vi "Calculator.vi"() -> ()   [LabVIEW 2013]
doc: "This VI is a fully-functional calculator built in LabVIEW. It demonstrates the following concepts taught in the LabVIEW Basics class.\n\n- Dataflow Programming\n- Modular Programming\n- While Loops\n- Shift Registers\n- Case Structures\n- Functional Global Variables\n- Event-Driven Programming\n- VI Documentation\n- Control/Indicator Documentation\n- Custom Controls/Type Definitions\n- LabVIEW Project and Application Builder\n\nAuthor: Erik Johnson, National Instruments"
panel:
  out "Output":string
  in  "Input":string
  in  "error in (no error)":errorcluster
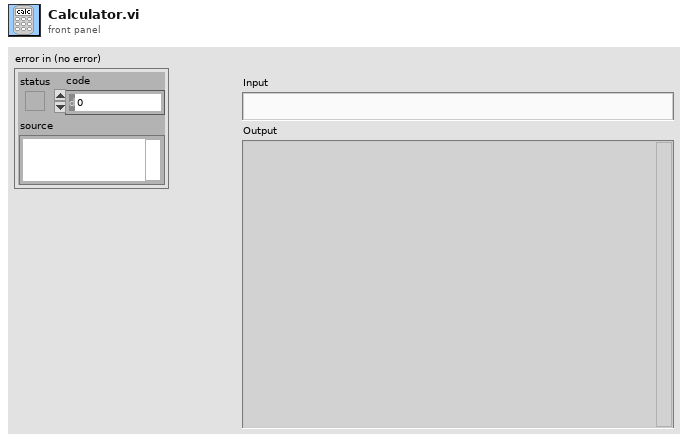
[diagram p1: front panel]
types:
  T1 = typedef "eventvkey.ctl" = enum16{"ASCII", "Enter", "Return", "Shift", "Ctrl", "Alt", "Cmd", "Opt", "Caps", "NumLock", "Clear", "Break", "Up", "Down", "Left", "Right", "Insert", "Delete", "Home", "End", "PageUp", "PageDown", "Escape", "Help", "Pause", "ScrollLock", "F1", "F2", "F3", "F4", "F5", "F6", "F7", "F8", "F9", "F10", "F11", "F12", "F13", "F14", "F15", "F16", "F17", "F18", "F19", "F20", "F21", "F22", "F23", "F24", "Play", "VolumeUp", "VolumeDown", "Mute", "Two Byte Char"}
  T2 = enum32{"invalid app kind", "Development System", "Run Time System", "Student Edition", "Embedded LabVIEW", "Evaluation", "Custom"}
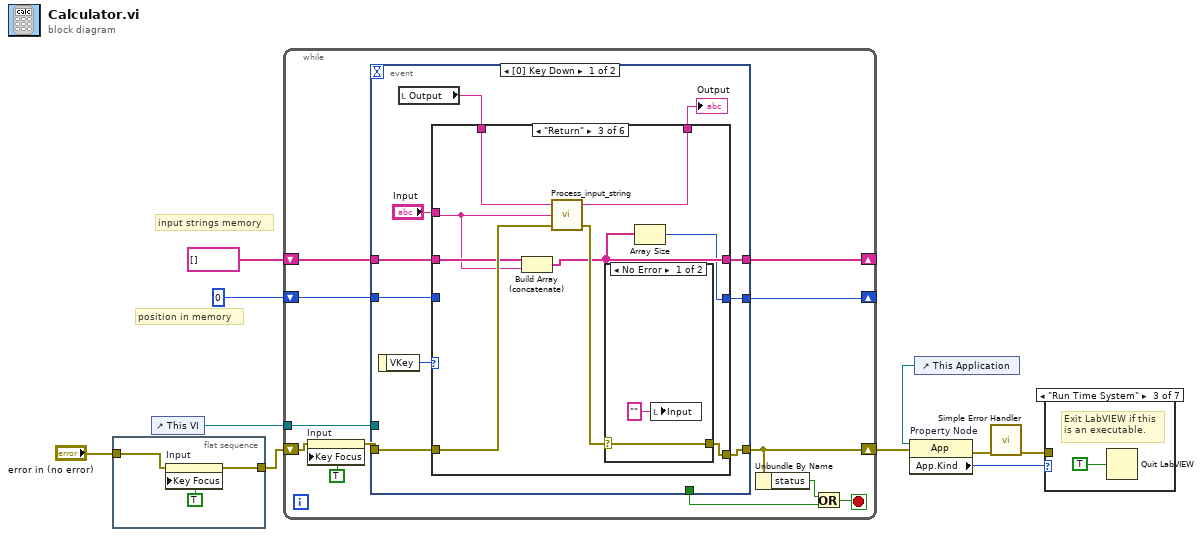
[diagram p0: block diagram]
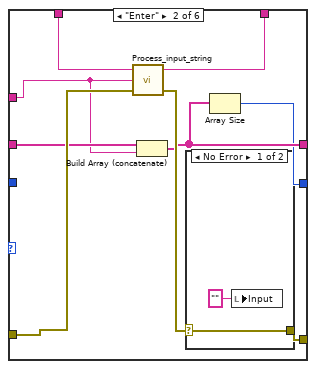
[diagram p9: hidden frame]
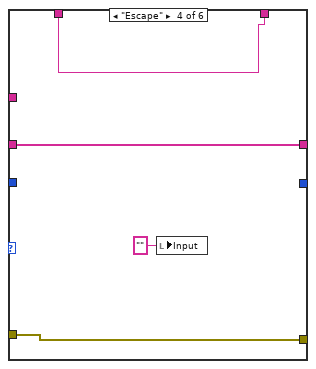
[diagram p12: hidden frame]
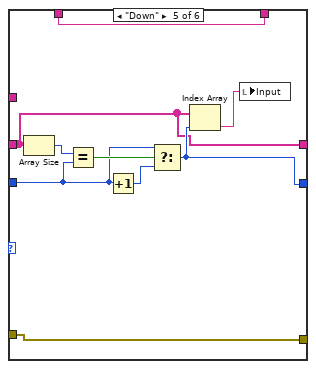
[diagram p13: hidden frame]
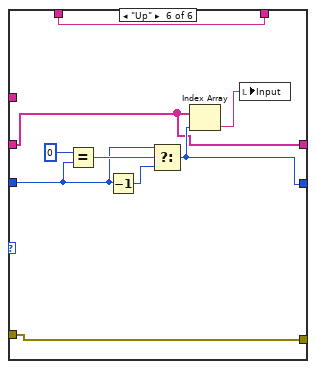
[diagram p14: hidden frame]
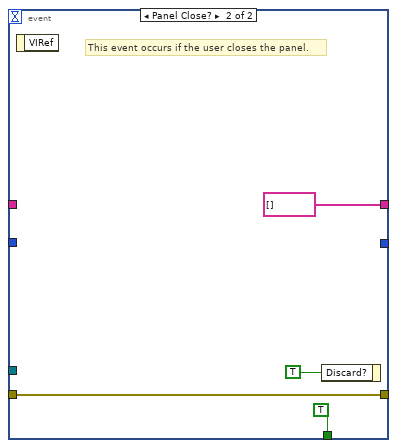
[diagram p15: hidden frame]
diagram:
  # "position in memory"
  # "input strings memory"
  n1 = flat-sequence {
    tunnel: "error in (no error)" -> [w12]
    tunnel: [w11] -> w1
    frame #0 {
      n2 = property on="Input" class="Str"(error in=w12, "Key Focus"=TRUE) -> (error out=w11:errorcluster)  [unwired: 1 in, 1 out]
    }
  }
  n3 = control-ref of="This VI"() -> (w5:refnum<vi>)
  n4 = while {
    tunnel: w5 -> [w25]
    shift-right: [w23] -> w6
    shift-left: w1 -> [w15]
    shift-right: [w19] -> _
    shift-left: string[] [] -> [w20]
    shift-right: [w17] -> _
    shift-left: 0 -> [w18]
    stop <- w24 stop-if-true
    n5 = property on="Input" class="Str"(error in=w15, "Key Focus"=TRUE) -> (error out=w14:errorcluster)  [unwired: 1 in, 1 out]
    n6 = event shown="[0] Key Down" {
      selector: _ -> [_ _]
      dyn-events: _ -> [_ _]
      timeout: _ -> [_ _]
      tunnel: [_ TRUE ("Discard?")] -> w21
      tunnel: w25 -> [_ _]
      tunnel: w14 -> [w31 w86]
      tunnel: [w30 w86] -> w23
      tunnel: w20 -> [w29 _]
      tunnel: [w28 string[] []] -> w19
      tunnel: w18 -> [w27 _]
      tunnel: [w26 _] -> w17
      event Key Down {
        n7 = event-data() -> ("VKey"=w35:T1)  [unwired: 1 in]
        n8 = local read "Output"() -> (w33:string)
        n9 = case shown="\"Return\"" w35 {
          tunnel: "Input" -> [_ w43 w55 _ _ _]
          tunnel: w33 -> [w38 w47 w58 w65 w68 w77]
          tunnel: [w38 w46 w59 w65 w68 w77] -> w32
          tunnel: w31 -> [w37 w45 w57 w64 w67 w76]
          tunnel: [w37 w41 w53 w64 w67 w76] -> w30
          tunnel: w29 -> [w36 w44 w56 w63 w69 w79]
          tunnel: [w36 w40 w52 w63 w69 w79] -> w28
          tunnel: w27 -> [_ _ _ _ w73 w83]
          tunnel: [_ w39 w51 _ w71 w81] -> w26
          frame "ASCII", Default {
          }
          frame "Enter" {
            n10 = call "Process_input_string.vi"("error in (no error)"=w45, "Input"=w43, "Output_window_old"=w47) -> ("error out"=w42:errorcluster, "Output"=w46:string)  [unwired: 1 out]
            n11 = Build Array (concatenate)(w44, w43) -> (w40:string[])
            n12 = case shown="No Error" w42 {
              selector: w42 -> [w49 w50]
              tunnel: [w49 w50] -> w41
              frame No Error {
                n13 = local write "Input"("" ("Input")) -> ()
              }
              frame Error {
              }
            }
            n14 = Array Size(array=w40) -> (size(s)=w39:i32)
          }
          frame "Return" {
            n15 = Build Array (concatenate)(w56, w55) -> (w52:string[])
            n16 = call "Process_input_string.vi"("error in (no error)"=w57, "Input"=w55, "Output_window_old"=w58) -> ("error out"=w54:errorcluster, "Output"=w59:string)  [unwired: 1 out]
            n17 = case shown="No Error" w54 {
              selector: w54 -> [w61 w62]
              tunnel: [w61 w62] -> w53
              frame No Error {
                n18 = local write "Input"("" ("Input")) -> ()
              }
              frame Error {
              }
            }
            n19 = Array Size(array=w52) -> (size(s)=w51:i32)
          }
          frame "Escape" {
            n20 = local write "Input"("" ("Input")) -> ()
          }
          frame "Down" {
            n21 = Array Size(array=w69) -> (size(s)=w75:i32)
            n22 = Equal?(x=w75, y=w73) -> (x = y?=w74:bool)
            n23 = Increment(x=w73) -> (x+1=w72:i32)
            n24 = Select(t=w73, s=w74, f=w72) -> (s? t:f=w71:i32)
            n25 = Index Array(array=w69, index=w71) -> (element=w70:string)
            n26 = local write "Input"(w70) -> ()
          }
          frame "Up" {
            n27 = Equal?(x=0, y=w83) -> (x = y?=w84:bool)
            n28 = Decrement(x=w83) -> (x-1=w82:i32)
            n29 = Select(t=w83, s=w84, f=w82) -> (s? t:f=w81:i32)
            n30 = Index Array(array=w79, index=w81) -> (element=w80:string)
            n31 = local write "Input"(w80) -> ()
          }
        }
        "Output" <- w32
      }
      event Panel Close? {
        # "This event occurs if the user closes the panel."
        n32 = event-data() -> ()  [unwired: 1 in, 1 out]
        n33 = event-data("Discard?"=TRUE) -> ()  [unwired: 1 in, 1 out]
      }
    }
    n34 = Unbundle By Name(w23) -> ("status"=w22:bool)
    n35 = Or(x=w22, y=w21) -> (x .or. y?=w24:bool)
  }
  n36 = control-ref of="This Application"() -> (w10:refnum<vi>)
  n37 = property on="Property Node" class="App"(reference=w10, error in=w6) -> (error out=w8:errorcluster, "App.Kind"=w9:T2)  [unwired: 1 out]
  n38 = call <vilib>:"Simple Error Handler.vi"("error in (no error)"=w8) -> ("error out"=w7:errorcluster)  [unwired: 4 in, 4 out]
  n39 = case shown="\"Run Time System\"" w9 {
    tunnel: w7 -> [_ _ _ _ _ _ _]
    frame "invalid app kind", Default {
    }
    frame "Development System" {
    }
    frame "Run Time System" {
      # "Exit LabVIEW if this\nis an executable."
      n40 = Quit LabVIEW(quit? (T)=TRUE) -> ()
    }
    frame "Student Edition" {
    }
    frame "Embedded LabVIEW" {
    }
    frame "Evaluation" {
    }
    frame "Custom" {
    }
  }
